vi "ReadBA6010.vi"(0 "VISA resource name 2":refnum<visa-resource-name>, 11 "error in (no error)":errorcluster) -> (4 "Resistance":dbl format="%.4g", 6 "Reactance":dbl format="%.4g", 8 "Capacitance":dbl format="%.4g", 10 "Dissipation Factor":dbl format="%.4g", 15 "error out":errorcluster)   [LabVIEW 2020]
doc: "Returns the actual voltage, current, and power level of the output."
panel:
  out "subarray 2":string[](array[string])
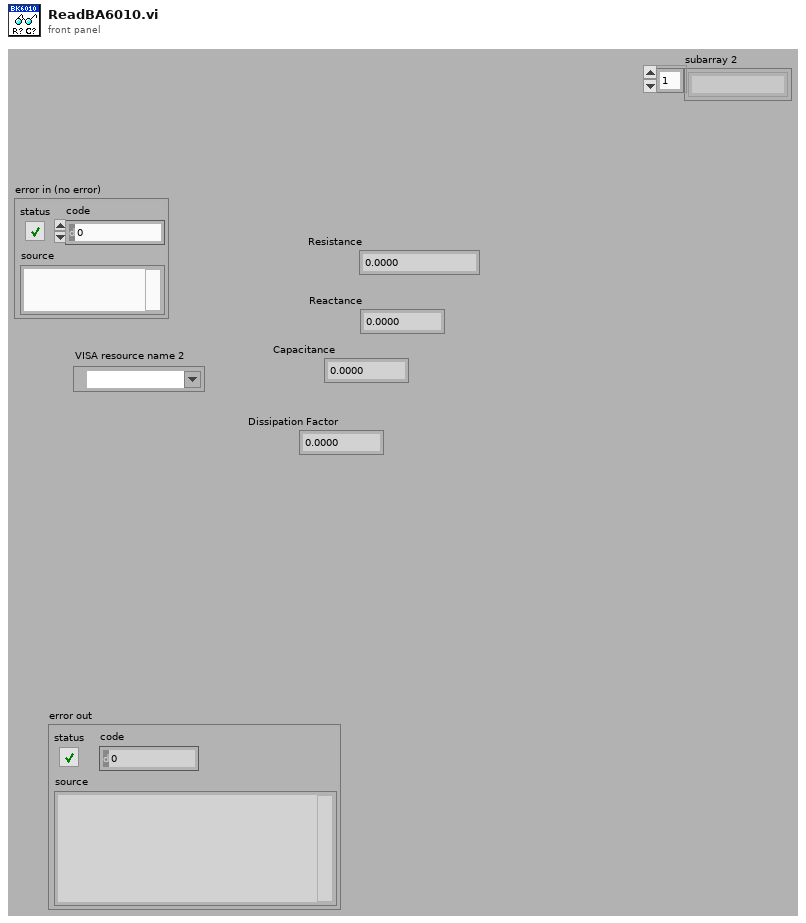
[diagram p1: front panel]
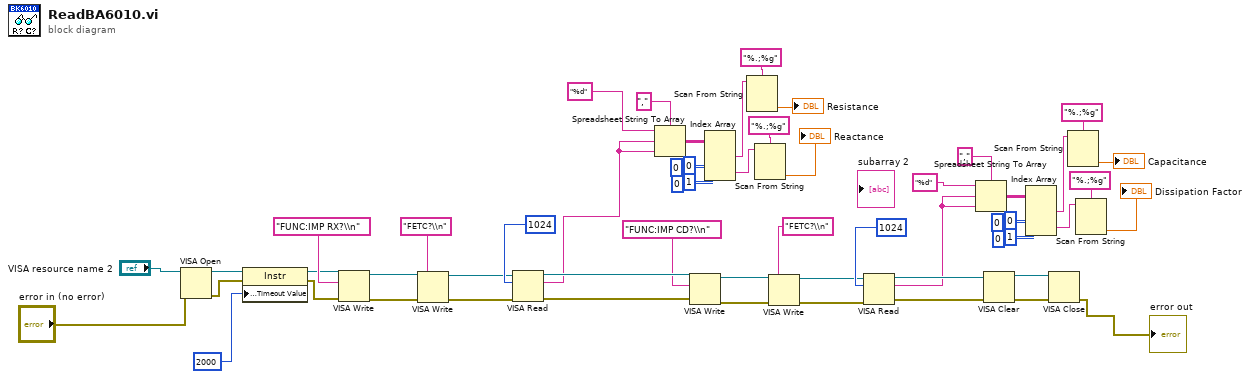
[diagram p0: block diagram]
diagram:
  n1 = VISA Open(error in (no error)="error in (no error)", VISA resource name="VISA resource name 2") -> (VISA resource name=w52:refnum<visa-resource-name>, error out=w51:errorcluster)  [unwired: 3 in]
  n2 = property class="Instr"(reference=w52, error in=w51, "General Settings:Timeout Value"=u32 2000) -> (reference out=w49:refnum<visa-resource-name>, error out=w50:errorcluster)
  n3 = VISA Write(VISA resource name=w49, write buffer="FUNC:IMP RX?\\n", error in (no error)=w50) -> (VISA resource name out=w41:refnum<visa-resource-name>, error out=w40:errorcluster)  [unwired: 1 out]
  n4 = VISA Write(VISA resource name=w41, write buffer="FETC?\\n", error in (no error)=w40) -> (VISA resource name out=w47:refnum<visa-resource-name>, error out=w46:errorcluster)  [unwired: 1 out]
  n5 = VISA Read(VISA resource name=w47, byte count=1024, error in (no error)=w46) -> (VISA resource name out=w33:refnum<visa-resource-name>, read buffer=w25:string, error out=w32:errorcluster)  [unwired: 1 out]
  n6 = Spreadsheet String To Array(delimiter (Tab)=",", format string="%d", spreadsheet string=w25, array type (2D Dbl)=w25) -> (array=w26:string[][])
  n7 = VISA Write(VISA resource name=w33, write buffer="FUNC:IMP CD?\\n", error in (no error)=w32) -> (VISA resource name out=w35:refnum<visa-resource-name>, error out=w34:errorcluster)  [unwired: 1 out]
  n8 = Index Array(array=w26, index (row) #1=0 ("disabled index (row)"), index (col) #1=0 ("disabled index (col)"), index (row) #2=0 ("disabled index (row)"), index (col) #2=1 ("index (col)")) -> (element #1=w15:string, element #2=w16:string)
  n9 = Scan From String(format string="%.;%g", input string=w15) -> (output 1=→"Resistance":dbl)  [unwired: 3 in, 3 out]
  n10 = Scan From String(format string="%.;%g", input string=w16) -> (output 1=→"Reactance":dbl)  [unwired: 3 in, 3 out]
  n11 = VISA Write(VISA resource name=w35, write buffer="FETC?\\n", error in (no error)=w34) -> (VISA resource name out=w38:refnum<visa-resource-name>, error out=w37:errorcluster)  [unwired: 1 out]
  n12 = VISA Read(VISA resource name=w38, byte count=1024, error in (no error)=w37) -> (VISA resource name out=w30:refnum<visa-resource-name>, read buffer=w3:string, error out=w29:errorcluster)  [unwired: 1 out]
  n13 = Spreadsheet String To Array(delimiter (Tab)=",", format string="%d", spreadsheet string=w3, array type (2D Dbl)=w3) -> (array=w12:string[][])
  n14 = VISA Clear(VISA resource name=w30, error in (no error)=w29) -> (VISA resource name out=w44:refnum<visa-resource-name>, error out=w43:errorcluster)
  n15 = Index Array(array=w12, index (row) #1=0 ("disabled index (row)"), index (col) #1=0 ("disabled index (col)"), index (row) #2=0 ("disabled index (row)"), index (col) #2=1 ("index (col)")) -> (element #1=w1:string, element #2=w2:string)
  n16 = VISA Close(VISA resource name=w44, error in (no error)=w43) -> (error out=→"error out":errorcluster)
  n17 = Scan From String(format string="%.;%g", input string=w1) -> (output 1=→"Capacitance":dbl)  [unwired: 3 in, 3 out]
  n18 = Scan From String(format string="%.;%g", input string=w2) -> (output 1=→"Dissipation Factor":dbl)  [unwired: 3 in, 3 out]
